vi "Scan Field str (SubVI).vi"(6 "字符串":string, 9 "queue out":refnum<queue>, 11 "队列输入":refnum<queue>) -> (0 "错误输出":errorcluster)   [LabVIEW 2019, in "Take Seq.lvlib"]
uses:
  Take Seq.lvlib
  config.ctl
  Instrument.ctl
  lib/QDInstrument.dll
  <vilib>/NI/Modbus Library/API/Master/Modbus Master.lvclass
  SubVI.lvlib
panel:
  # "(真是通道1，假是通道2)"
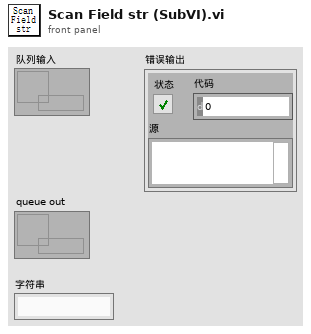
[diagram p1: front panel]
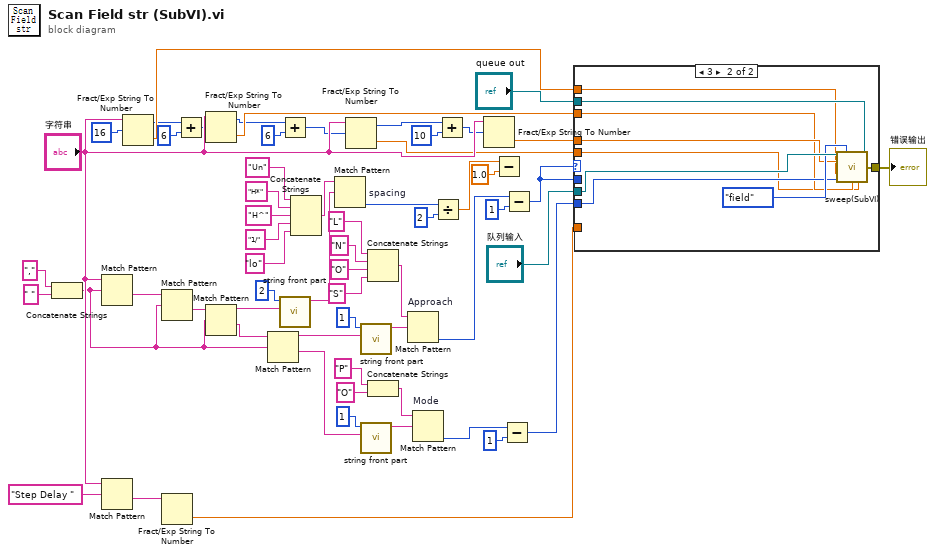
[diagram p0: block diagram]
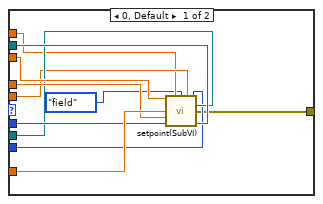
[diagram p2: hidden frame]
diagram:
  n1 = Concatenate Strings("," ("字符串"), " " ("字符串")) -> (w43:string)
  n2 = Match Pattern(string="字符串", regular expression=w43) -> (after substring=w1:string)  [unwired: 1 in, 3 out]
  n3 = Match Pattern(string="字符串", regular expression="Step Delay ") -> (after substring=w57:string)  [unwired: 1 in, 3 out]
  n4 = Fract/Exp String To Number(string="字符串", offset=16 ("偏移量")) -> (offset past number=w3:i32, number=w51:dbl)  [unwired: 2 in]
  n5 = Match Pattern(string=w1, regular expression=w43) -> (after substring=w27:string)  [unwired: 1 in, 3 out]
  n6 = Fract/Exp String To Number(string=w57) -> (number=w58:dbl)  [unwired: 3 in, 1 out]
  n7 = Add(x=w3, y=6) -> (x+y=w4:i32)
  n8 = Fract/Exp String To Number(string="字符串", offset=w4) -> (offset past number=w22:i32, number=w50:dbl)  [unwired: 2 in]
  n9 = Match Pattern(string=w27, regular expression=w43) -> (before substring=w28:string, after substring=w42:string)  [unwired: 1 in, 2 out]
  n10 = Match Pattern(string=w42, regular expression=w43) -> (before substring=w44:string, after substring=w45:string)  [unwired: 1 in, 2 out]
  n11 = Add(x=w22, y=6) -> (x+y=w24:i32)
  n12 = call "string front part.vi"("字符串"=w28, "偏移量(0)"=2) -> ("result string"=w30:string)  [unwired: 9 in]
  n13 = Concatenate Strings("Un" ("字符串"), "H*" ("字符串"), "H^" ("字符串"), "1/" ("字符串"), "lo" ("字符串")) -> (w36:string)
  n14 = Match Pattern "spacing"(string=w36, regular expression=w30) -> (offset past match=w37:i32)  [unwired: 1 in, 3 out]
  n15 = Fract/Exp String To Number(string="字符串", offset=w24) -> (offset past number=w41:i32, number=w52:dbl)  [unwired: 2 in]
  n16 = call "string front part.vi"("字符串"=w44, "偏移量(0)"=1) -> ("result string"=w7:string)  [unwired: 9 in]
  n17 = call "string front part.vi"("字符串"=w45, "偏移量(0)"=1) -> ("result string"=w14:string)  [unwired: 9 in]
  n18 = Concatenate Strings("L" ("字符串"), "N" ("字符串"), "O" ("字符串"), "S" ("字符串")) -> (w11:string)
  n19 = Concatenate Strings("P" ("字符串"), "O" ("字符串")) -> (w17:string)
  n20 = Match Pattern "Approach"(string=w11, regular expression=w7) -> (offset past match=w46:i32)  [unwired: 1 in, 3 out]
  n21 = Match Pattern "Mode"(string=w17, regular expression=w14) -> (offset past match=w18:i32)  [unwired: 1 in, 3 out]
  n22 = Divide(x=w37, y=2) -> (x/y=w39:dbl)
  n23 = Add(x=w41, y=10) -> (x+y=w26:i32)
  n24 = Fract/Exp String To Number(string="字符串", offset=w26) -> (number=w49:dbl)  [unwired: 2 in, 1 out]
  n25 = Subtract(x=w39, y=1.0) -> ()  [unwired: 1 out]
  n26 = Subtract(x=w18, y=1) -> (x-y=w48:i32)
  n27 = Subtract(x=w46, y=1) -> (x-y=w54:i32)
  n28 = case shown="3" w54 {
    tunnel: w48 -> [w65 w75]
    tunnel: w54 -> [w68 _]
    tunnel: w49 -> [w69 w77]
    tunnel: w50 -> [w71 w74]
    tunnel: w51 -> [w63 w76]
    tunnel: w52 -> [w64 w73]
    tunnel: "队列输入" -> [w66 w80]
    tunnel: "queue out" -> [w67 w79]
    tunnel: [w61 w72] -> w56
    tunnel: w58 -> [w70 _]
    frame 0, Default {
      n29 = call "setpoint(SubVI).vi"("Filed 2"=w71, "Field"=w63, "类型"=enum16{"temp", "field", "position"}."field", "Rate/speed"=w64, "Mode"=w65, "data"=w66, "Delay"=w70, "steps number"=w69, "Approach"=w68, "config"=w67) -> ("错误输出"=w61:errorcluster)  [unwired: 5 in]
    }
    frame 3 {
      n30 = call "sweep(SubVI).vi"("data"=w80, "类型"=enum16{"temp", "field", "position"}."field", "config"=w79, "steps number"=w77, "Field"=w76, "Mode"=w75, "Field 2"=w74, "Rate、speed"=w73) -> ("错误输出"=w72:errorcluster)  [unwired: 7 in]
    }
  }
  "错误输出" <- w56
